vi "Read Ai.vi"(0 "FPGA API in":refnum<class "FPGA API.lvclass">, 11 "error in (no error)":errorcluster) -> (4 "FPGA API out":refnum<class "FPGA API.lvclass">, 6 "AI Data":dbl[][](array[numeric]), 8 "Valud Data":bool, 15 "error out":errorcluster)   [LabVIEW 2019, in "FPGA API.lvclass"]
uses:
  FPGA API.lvclass
  FPGA API.lvclass/FPGA API.ctl
  <vilib>/Utility/error.llb/Error Cluster From Error Code.vi
  <vilib>/rvi/errors/niLvFpgaAdjustHostInterfaceError.vi
  <vilib>/rvi/interface/nirviMethod/nirviMethod.xnode
  FPGA Ref.ctl
  <vilib>/FPGAPlugInAG/Dynamic/niLvFpga_ReadFifo_Dynamic.vi
  <vilib>/rvi/errors/niLvFpgaMergeErrorWithErrorCode.vi
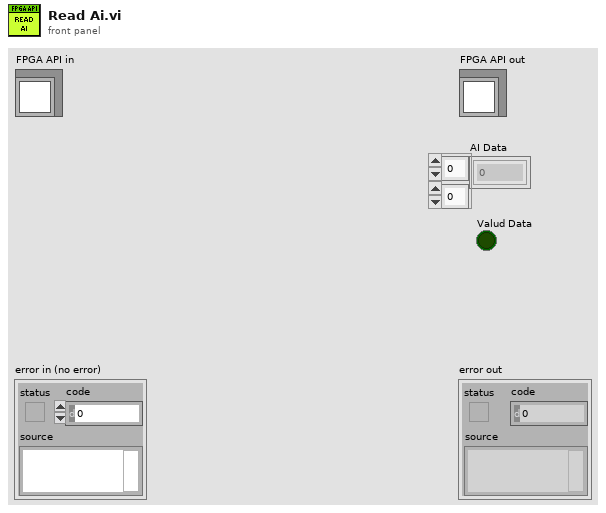
[diagram p1: front panel]
types:
  T1 = typedef "FPGA API.lvclass/FPGA Ref.ctl" = refnum<k20>
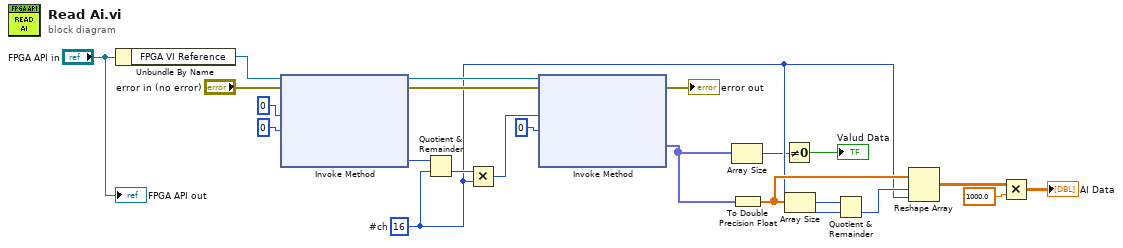
[diagram p0: block diagram]
diagram:
  w6 = u32 16  # #ch
  n1 = Unbundle By Name("FPGA API in") -> ("FPGA VI Reference"=w20:T1)
  n2 = xnode "Invoke Method"("FPGA VI Reference In"=w20, "error in"="error in (no error)", "Number of Elements"=u32 0, "Timeout (ms)"=0) -> ("FPGA VI Reference Out"=w15:T1, "error out"=w16:errorcluster, "Elements Remaining"=w17:u32)  [unwired: 1 out]
  n3 = Quotient & Remainder(x=w17, y=w6) -> (floor(x/y)=w13:u32)  [unwired: 1 out]
  n4 = Multiply(x=w13, y=w6) -> (x*y=w11:u32)
  n5 = xnode "Invoke Method"("FPGA VI Reference In"=w15, "error in"=w16, "Number of Elements"=w11, "Timeout (ms)"=0) -> ("error out"=→"error out":errorcluster, "Data"=w4:fxp<+/-,21,-4>[])  [unwired: 2 out]
  n6 = Array Size(array=w4) -> (size(s)=w3:i32)
  n7 = To Double Precision Float(number=w4) -> (double precision float=w7:dbl[])
  n8 = Not Equal To 0?(x=w3) -> (x != 0?=→"Valud Data":bool)
  n9 = Array Size(array=w7) -> (size(s)=w9:i32)
  n10 = Quotient & Remainder(x=w9, y=w6) -> (floor(x/y)=w8:u32)  [unwired: 1 out]
  n11 = Reshape Array(w7, w8, w6) -> (w5:dbl[][])
  n12 = Multiply(x=w5, y=1000.0) -> (x*y=→"AI Data":dbl[][])
  "FPGA API out" <- "FPGA API in"
